vi "HeapFree.vi"(4 "error in (no error)":errorcluster, 5 "HEAP_NO_SERIALIZE":bool, 6 "lpMem (NULL)":i32, 7 "hHeap (NULL)":i32) -> (0 "error out":errorcluster, 3 "dup hHeap":i32)   [LabVIEW 2011]
uses:
  KERNEL32.DLL
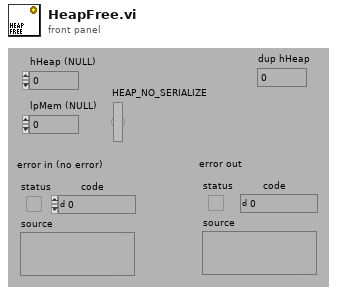
[diagram p1: front panel]
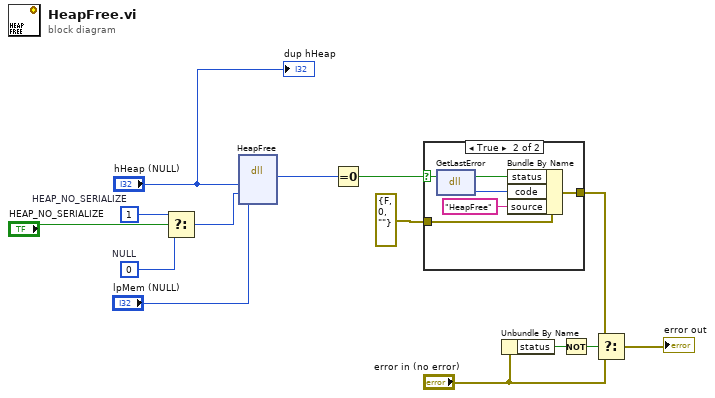
[diagram p0: block diagram]
diagram:
  w3 = u32 0  # NULL
  w5 = u32 1  # HEAP_NO_SERIALIZE
  n1 = Select(t=w5, s="HEAP_NO_SERIALIZE", f=w3) -> (s? t:f=w2:u32)
  n2 = dll-call lib="KERNEL32.DLL" fn="HeapFree" label="BOOL HeapFree(\n  HANDLE hHeap,  // handle to heap\n  DWORD dwFlags, // heap free options\n  LPVOID lpMem   // pointer to memory\n);"("hHeap"="hHeap (NULL)", "dwFlags"=w2, "lpMem"="lpMem (NULL)") -> ("lpMem"=w8:i32)  [unwired: 6 in, 2 out]
  n3 = Equal To 0?(x=w8) -> (x = 0?=w7:bool)
  n4 = case shown="True" w7 {
    selector: w7 -> [_ w18]
    tunnel: [w15 w19] -> w12
    tunnel: errorcluster {"status"=FALSE, "code"=0, "source"=""} ("error out") -> [w15 w17]
    frame False {
    }
    frame True {
      n5 = dll-call lib="KERNEL32.DLL" fn="GetLastError"() -> (w16:i32)  [unwired: 3 in, 2 out]
      n6 = Bundle By Name(cluster=w17, "status"=w18, "code"=w16, "source"="HeapFree") -> (w19:errorcluster)
    }
  }
  n7 = Unbundle By Name("error in (no error)") -> ("status"=w13:bool)
  n8 = Not(x=w13) -> (.not. x?=w10:bool)
  n9 = Select(t=w12, s=w10, f="error in (no error)") -> (s? t:f=→"error out":errorcluster)
  "dup hHeap" <- "hHeap (NULL)"
